vi "DAQmx Read (Digital Bool 1Line 1Point).vi"(0 "task/channels in":refnum<k21>, 9 "timeout":dbl=10.0 format="%0.2f", 11 "error in":errorcluster) -> (4 "task out":refnum<k21>, 6 "data":bool, 15 "error out":errorcluster)   [LabVIEW 2011]
doc: "Reads a single Boolean sample from a task that contains a digital input channel composed of a single line."
uses:
  nilvaiu.dll
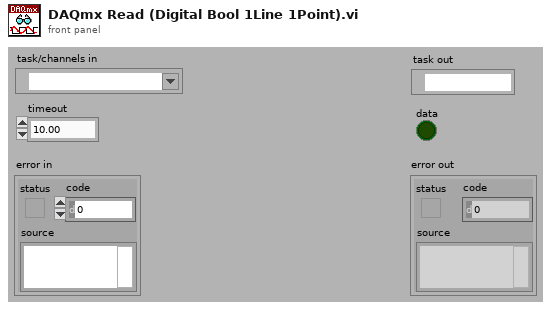
[diagram p1: front panel]
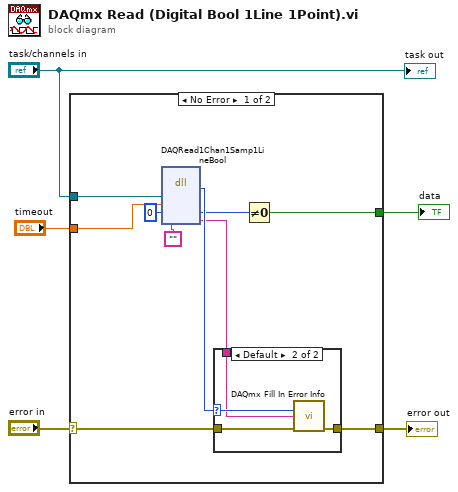
[diagram p0: block diagram]
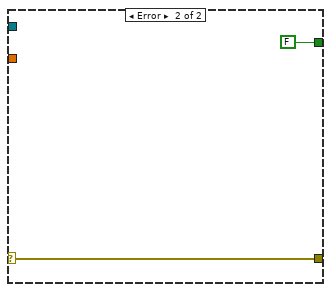
[diagram p3: hidden frame]
diagram:
  n1 = case shown="No Error" "error in" {
    selector: "error in" -> [w7 w21]
    tunnel: [w13 w21] -> w4
    tunnel: "task/channels in" -> [w15 _]
    tunnel: [w8 FALSE] -> w2
    tunnel: "timeout" -> [w6 _]
    frame No Error {
      n2 = dll-call lib="nilvaiu.*" fn="DAQRead1Chan1Samp1LineBool"("taskID"=w15, "timeout"=w6, "data"=u8 0, "extendedErrorInfo"="") -> (w14:i32, "data"=w10:u8, "extendedErrorInfo"=w11:string)  [unwired: 4 in, 3 out]
      n3 = case shown="Default" w14 {
        selector: w14 -> [_ w19]
        tunnel: w7 -> [w16 w20]
        tunnel: [w16 w18] -> w13
        tunnel: w11 -> [_ w17]
        frame 0 {
        }
        frame Default {
          n4 = call "DAQmx Fill In Error Info.vi"("status code"=w19, "extended error info"=w17, "error in"=w20) -> ("error out"=w18:errorcluster)  [unwired: 1 in, 11 out]
        }
      }
      n5 = Not Equal To 0?(x=w10) -> (x != 0?=w8:bool)
    }
    frame Error {
    }
  }
  "error out" <- w4
  "data" <- w2
  "task out" <- "task/channels in"
